vi "sendCmdStatus.vi"(8 "error in (no error)":errorcluster, 9 "cmdStatus":string(combo)="ack", 10 "packet":string, 11 "tcpServer in":refnum<class "TcpServer.lvclass">) -> (0 "error out":errorcluster, 3 "tcpServer out":refnum<class "TcpServer.lvclass">)   [LabVIEW 2018, in "TcpServer.lvclass"]
doc: "Send cmdStatus to the TCP Server to inform the TCP Client about the command result."
uses:
  TcpServer.lvclass
  TcpServerCmd/typedef/ackTypeDef.ctl
  TcpServer.lvclass/TcpServer.ctl
  TcpServerCmd/TcpServerCmd.lvclass/TcpServerCmd.ctl
  TcpServerCmd/TcpServerCmd.lvclass
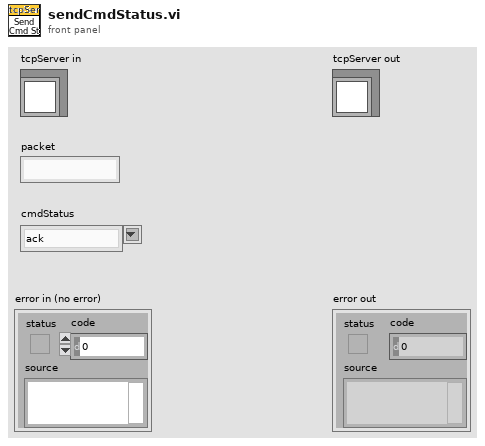
[diagram p1: front panel]
types:
  T1 = typedef "TcpServerCmd.lvclass/ackTypeDef.ctl" = cluster{"packet":string, "cmdStatus":string}
  T2 = typedef "TcpServerCmd.lvclass/userEventTypeDef.ctl" = cluster{"CmdRead":refnum<user-event>, "CmdWrite":refnum<user-event>, "EvtRead":refnum<user-event>, "EvtWrite":refnum<user-event>, "GenRead":refnum<user-event>, "GenWrite":refnum<user-event>}
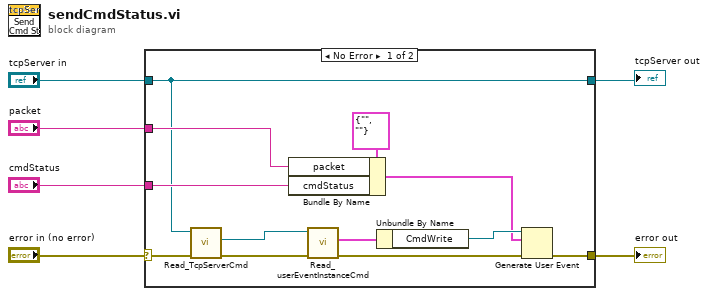
[diagram p0: block diagram]
diagram:
  n1 = case shown="No Error" "error in (no error)" {
    selector: "error in (no error)" -> [w9 w20]
    tunnel: [w17 w20] -> w5
    tunnel: "cmdStatus" -> [w18 _]
    tunnel: "packet" -> [w16 _]
    tunnel: "tcpServer in" -> [w7 w19]
    tunnel: [w7 w19] -> w1
    frame No Error {
      n2 = call "Read_TcpServerCmd.vi"("error in (no error)"=w9, "TcpServer in"=w7) -> ("error out"=w13:errorcluster, "TcpServerCmd.lvclass"=w14:refnum<class "TcpServerCmd.lvclass">)  [unwired: 7 in, 1 out]
      n3 = Bundle By Name(cluster=T1 {"packet"="", "cmdStatus"=""} ("ack"), "packet"=w16, "cmdStatus"=w18) -> (w10:T1)
      n4 = call "Read_userEventInstanceCmd.vi"("error in (no error)"=w13, "TcpServerCmd in"=w14) -> ("error out"=w8:errorcluster, "userEventInstance"=w12:T2)  [unwired: 7 in, 1 out]
      n5 = Unbundle By Name(w12) -> ("CmdWrite"=w11:refnum<user-event>)
      n6 = Generate User Event(user event=w11, event data cluster=w10, error in=w8) -> (error out=w17:errorcluster)  [unwired: 1 in, 1 out]
    }
    frame Error {
    }
  }
  "error out" <- w5
  "tcpServer out" <- w1
